vi "Generic_Detail_Window.vi"() -> ()   [LabVIEW 2018]
uses:
  <vilib>/Utility/miscctls.llb/LVPointTypeDef.ctl
panel:
  out "Storage Medium":string
  out "AC Connection":string
  out "Storage Capacity":dbl
  out "Nominal Power":dbl
  out "Device 2 Picture":u16(ring)
  out "Device 1 Picture":u16(ring)
  out "Label":string
  out "Device 2 Logo":u16(ring)
  out "Device 1 Logo":u16(ring)
  out "String":string="DER0"
  in  "Close":bool
  out "DER":i32
  out "Display Cluster":cluster{"DER":i32}
  out "Event":refnum<user-event>
  out "DER Names":string[](array[string])
  out "Storage Capacity Vector":dbl[](array[numeric])
  out "Storage Medium Vector":string[](array[string])
  out "Nominal Power Vector":dbl[](array[numeric])
  out "AC Connection Vector":string[](array[string])
  # "Information"
  # "DER:"
  # "Device 1"
  # "Characteristics"
  # "Nominal Power:"
  # "kW"
  # "Storage Capacity:"
  # "kWh"
  # "Storage Medium:"
  # "AC Connection:"
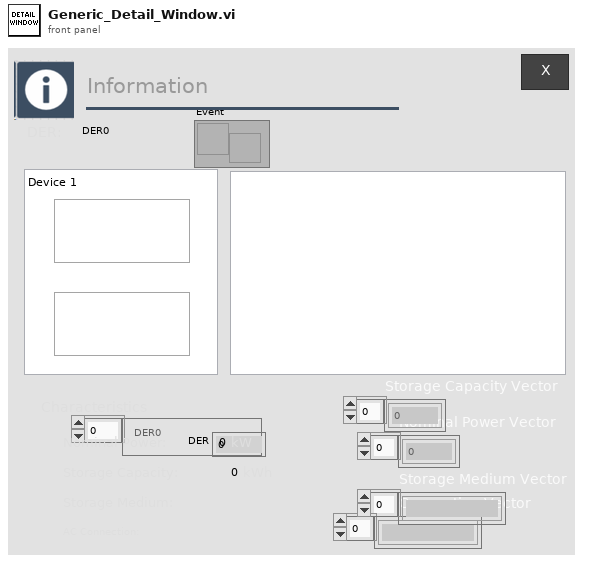
[diagram p1: front panel]
types:
  T1 = typedef "LVPointTypeDef.ctl" = cluster{"Horizontal":i16, "Vertical":i16}
  T2 = enum32{"Invalid", "Default", "Floating", "Floating/Auto-Hide", "Modal"}
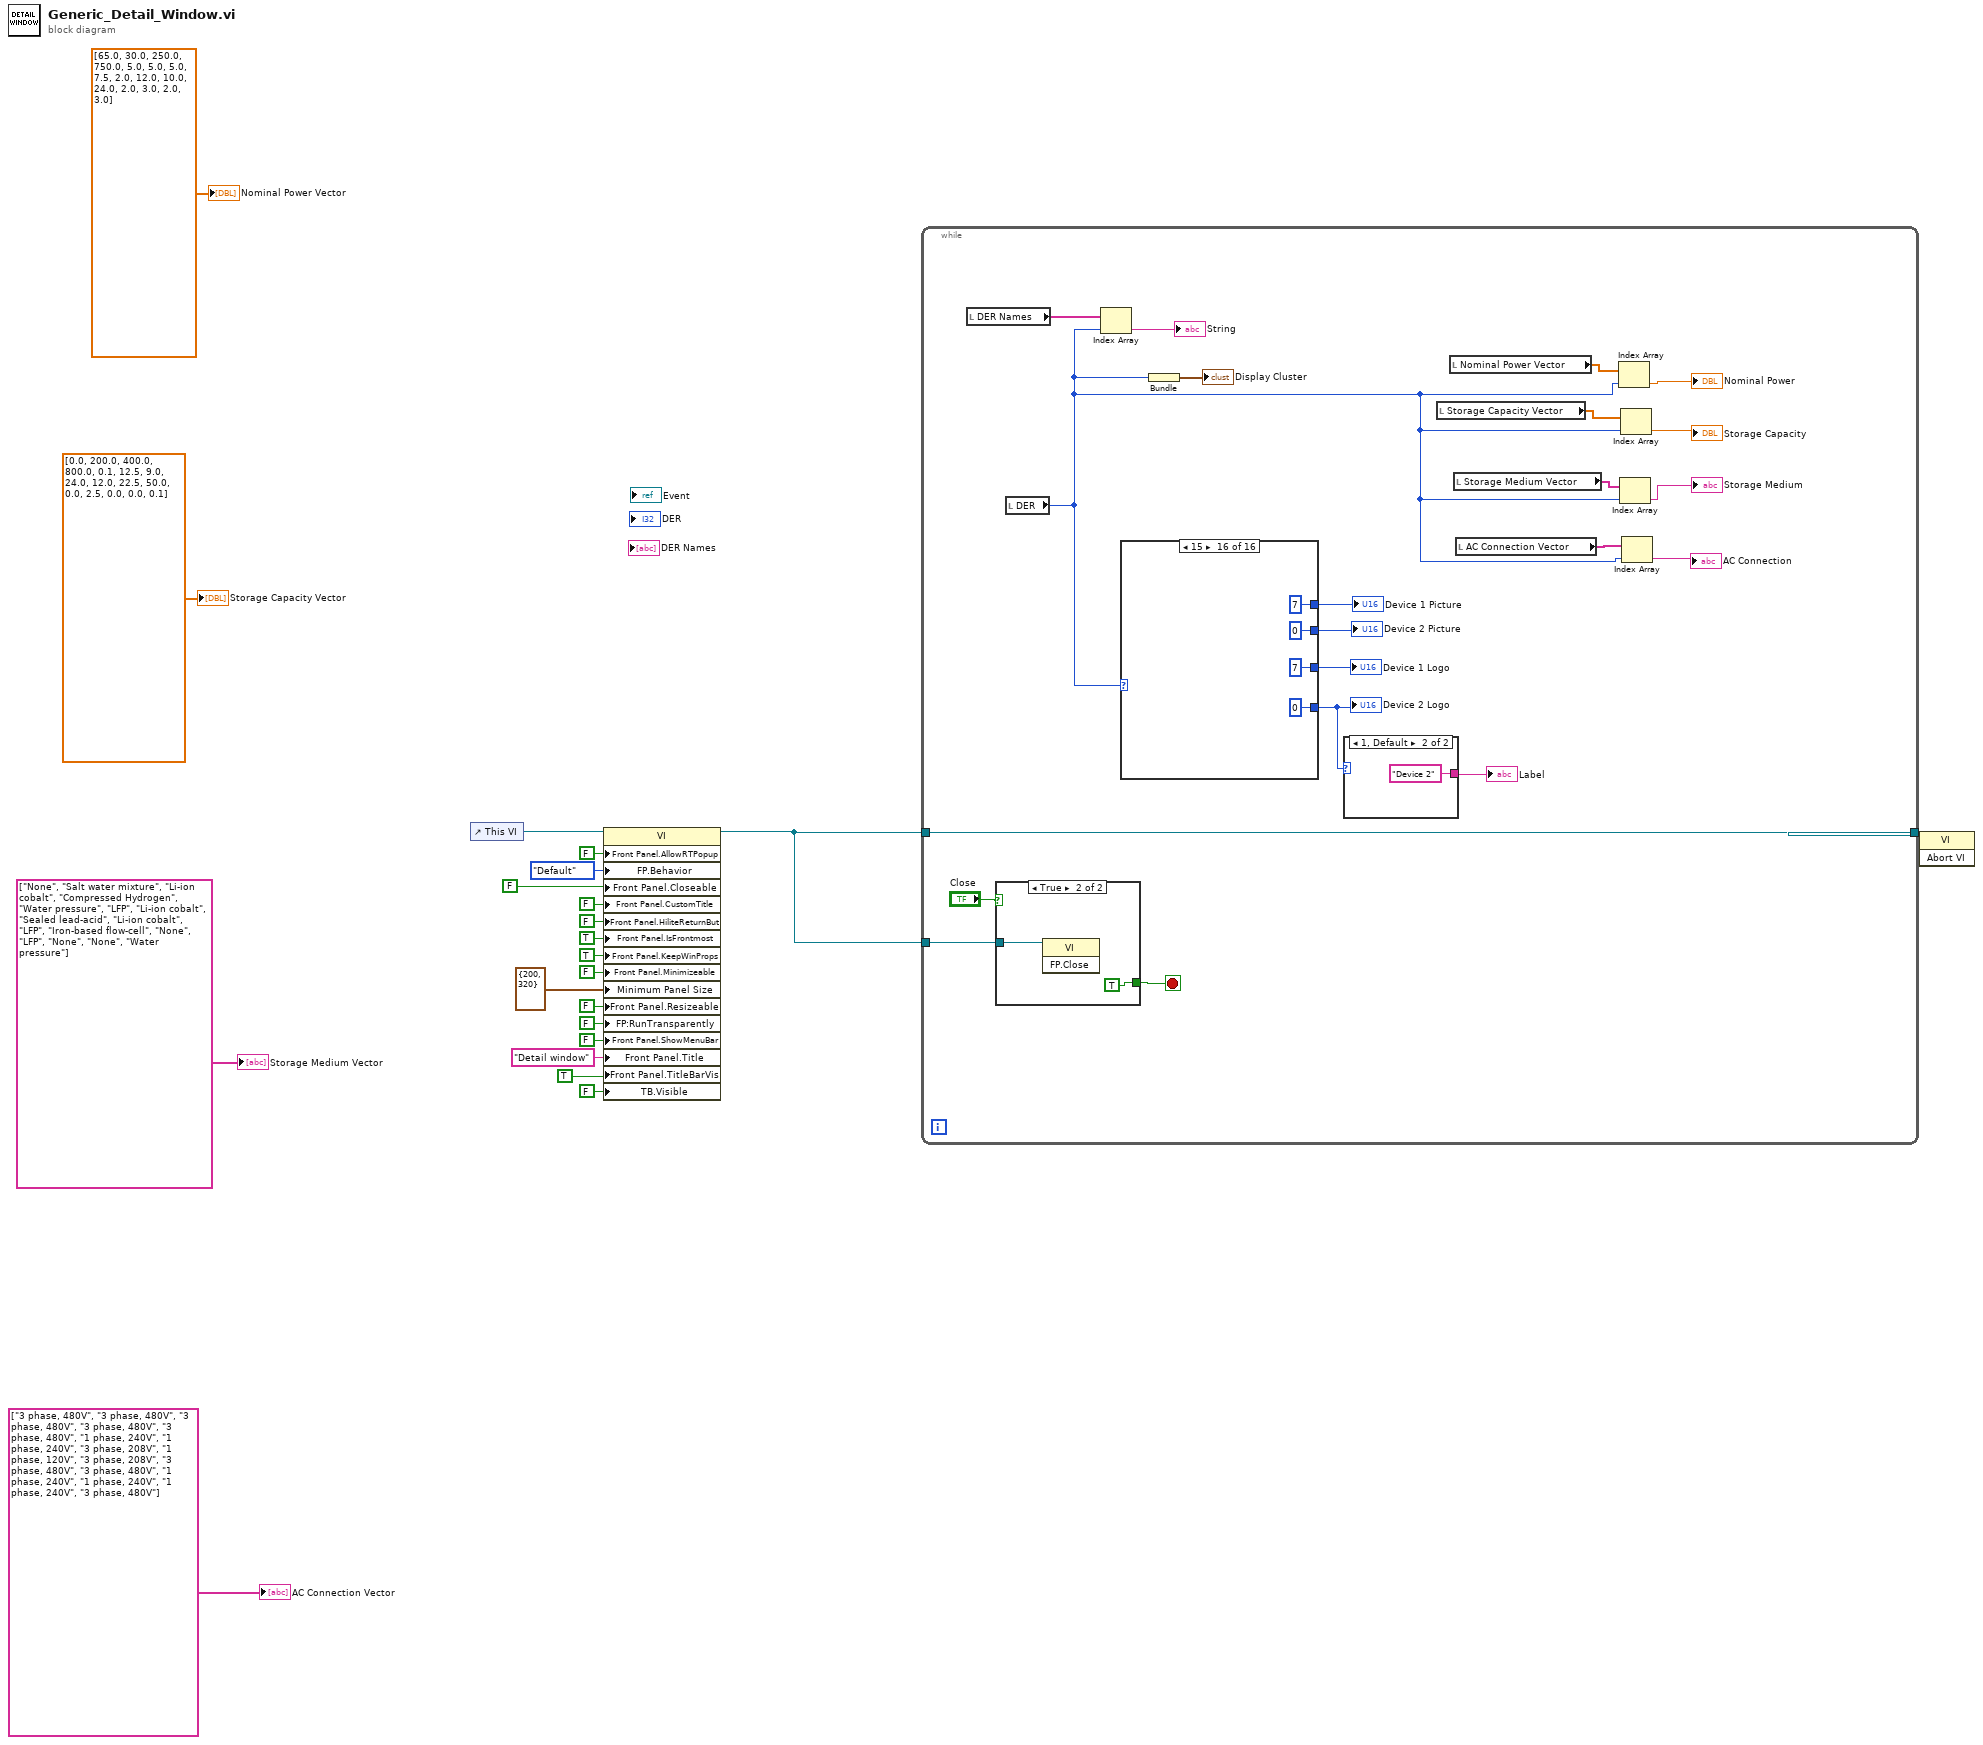
[diagram p0: block diagram]
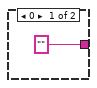
[diagram p2: hidden frame]
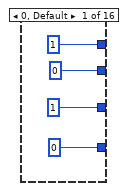
[diagram p3: hidden frame]
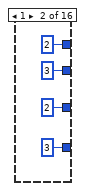
[diagram p4: hidden frame]
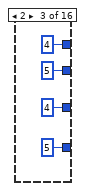
[diagram p5: hidden frame]
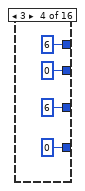
[diagram p6: hidden frame]
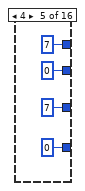
[diagram p7: hidden frame]
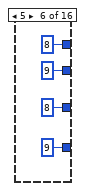
[diagram p8: hidden frame]
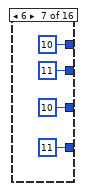
[diagram p9: hidden frame]
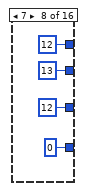
[diagram p10: hidden frame]
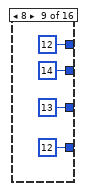
[diagram p11: hidden frame]
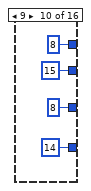
[diagram p12: hidden frame]
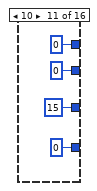
[diagram p13: hidden frame]
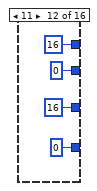
[diagram p14: hidden frame]
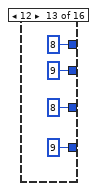
[diagram p15: hidden frame]
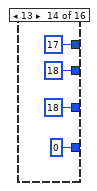
[diagram p16: hidden frame]
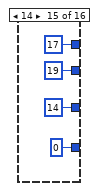
[diagram p17: hidden frame]
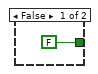
[diagram p18: hidden frame]
diagram:
  n1 = control-ref of="This VI"() -> (w22:refnum<vi>)
  n2 = property class="VI"(reference=w22, "Front Panel.AllowRTPopup"=FALSE ("Front Panel Window:Allow Runtime PopUp"), "FP.Behavior"=T2."Default" ("Front Panel Window:Behavior"), "Front Panel.Closeable"=FALSE ("Front Panel Window:Closeable"), "Front Panel.CustomTitle"=FALSE ("Front Panel Window:Custom Title"), "Front Panel.HiliteReturnBut"=FALSE ("Front Panel Window:Highlight Return Button"), "Front Panel.IsFrontmost"=TRUE ("Front Panel Window:Is Frontmost"), "Front Panel.KeepWinProps"=TRUE ("Front Panel Window:Keep Window Proportions"), "Front Panel.Minimizeable"=FALSE ("Front Panel Window:Minimizable"), "Minimum Panel Size"=T1 {"Horizontal"=200, "Vertical"=320} ("Front Panel Window:Minimum Size"), "Front Panel.Resizeable"=FALSE ("Front Panel Window:Resizable"), "FP:RunTransparently"=FALSE ("Front Panel Window:Run VI Transparently"), "Front Panel.ShowMenuBar"=FALSE ("Front Panel Window:Show Menu Bar"), "Front Panel.Title"="Detail window" ("Front Panel Window:Title"), "Front Panel.TitleBarVis"=TRUE ("Front Panel Window:Title Bar Visible"), "TB.Visible"=FALSE ("Tool Bar:Visible")) -> (reference out=w6:refnum<vi>)  [unwired: 1 in, 1 out]
  n3 = while {
    tunnel: w6 -> [w42]
    tunnel: [w40] -> w5
    tunnel: w6 -> [w40]
    stop <- w41 stop-if-true
    n4 = local read "DER Names"() -> (w39:string[])
    n5 = case shown="True" "Close" {
      tunnel: w42 -> [_ w112]
      tunnel: [FALSE TRUE] -> w41
      frame False {
      }
      frame True {
        n6 = invoke class="VI" method="FP.Close"(reference=w112) -> ()  [unwired: 2 in, 3 out]
      }
    }
    n7 = local read "DER"() -> (w26:i32)
    n8 = Index Array(array=w39, index=w26) -> (element=→"String":string)
    n9 = case shown="15" w26 {
      tunnel: [u16 1 u16 2 u16 4 u16 6 u16 7 u16 8 u16 10 u16 12 u16 13 u16 8 u16 15 u16 16 u16 8 u16 18 u16 14 u16 7] -> w36
      tunnel: [u16 0 u16 3 u16 5 u16 0 u16 0 u16 9 u16 11 u16 0 u16 12 u16 14 u16 0 u16 0 u16 9 u16 0 u16 0 u16 0] -> w35
      tunnel: [u16 1 u16 2 u16 4 u16 6 u16 7 u16 8 u16 10 u16 12 u16 12 u16 8 u16 0 u16 16 u16 8 u16 17 u16 17 u16 7] -> w33
      tunnel: [u16 0 u16 3 u16 5 u16 0 u16 0 u16 9 u16 11 u16 13 u16 14 u16 15 u16 0 u16 0 u16 9 u16 18 u16 19 u16 0] -> w32
      frame 0, Default {
      }
      frame 1 {
      }
      frame 2 {
      }
      frame 3 {
      }
      frame 4 {
      }
      frame 5 {
      }
      frame 6 {
      }
      frame 7 {
      }
      frame 8 {
      }
      frame 9 {
      }
      frame 10 {
      }
      frame 11 {
      }
      frame 12 {
      }
      frame 13 {
      }
      frame 14 {
      }
      frame 15 {
      }
    }
    "Device 1 Logo" <- w36
    "Device 2 Logo" <- w35
    "Device 1 Picture" <- w33
    "Device 2 Picture" <- w32
    n10 = Bundle("DER"=w26) -> (→"Display Cluster":cluster{"DER":i32})  [unwired: 1 in]
    n11 = case shown="1, Default" w35 {
      tunnel: ["" ("Label") "Device 2" ("Label")] -> w34
      frame 0 {
      }
      frame 1, Default {
      }
    }
    "Label" <- w34
    n12 = local read "Storage Capacity Vector"() -> (w29:dbl[])
    n13 = local read "Nominal Power Vector"() -> (w30:dbl[])
    n14 = local read "Storage Medium Vector"() -> (w28:string[])
    n15 = local read "AC Connection Vector"() -> (w27:string[])
    n16 = Index Array(array=w30, index=w26) -> (element=→"Nominal Power":dbl)
    n17 = Index Array(array=w28, index=w26) -> (element=→"Storage Medium":string)
    n18 = Index Array(array=w29, index=w26) -> (element=→"Storage Capacity":dbl)
    n19 = Index Array(array=w27, index=w26) -> (element=→"AC Connection":string)
  }
  n20 = invoke class="VI" method="Abort VI"(reference=w5) -> ()  [unwired: 2 in, 3 out]
  "Nominal Power Vector" <- dbl[] [65.0, 30.0, 250.0, 750.0, 5.0, 5.0, 5.0, 7.5, 2.0, 12.0, 10.0, 24.0, 2.0, 3.0, 2.0, 3.0]
  "Storage Capacity Vector" <- dbl[] [0.0, 200.0, 400.0, 800.0, 0.1, 12.5, 9.0, 24.0, 12.0, 22.5, 50.0, 0.0, 2.5, 0.0, 0.0, 0.1]
  "Storage Medium Vector" <- string[] ["None", "Salt water mixture", "Li-ion cobalt", "Compressed Hydrogen", "Water pressure", "LFP", "Li-ion cobalt", "Sealed lead-acid", "Li-ion cobalt", "LFP", "Iron-based flow-cell", "None", "LFP", "None", "None", "Water pressure"]
  "AC Connection Vector" <- string[] ["3 phase, 480V", "3 phase, 480V", "3 phase, 480V", "3 phase, 480V", "3 phase, 480V", "1 phase, 240V", "1 phase, 240V", "3 phase, 208V", "1 phase, 120V", "3 phase, 208V", "3 phase, 480V", "3 phase, 480V", "1 phase, 240V", "1 phase, 240V", "1 phase, 240V", "3 phase, 480V"]
